vi "Loader.vi"(8 "error in (no error)":errorcluster, 10 "Path":path, 11 "Config_Read.lvclass":refnum<class "Config_Read_BML.lvclass">) -> (0 "error out":errorcluster, 1 "Pattern_Name":string, 2 "FRM_Data_Array":T1[](array[typedef]) {"Data" format="%x"; "Start_Addr" format="%x"}, 3 "Config_Read.lvclass out":refnum<class "Config_Read_BML.lvclass">)   [LabVIEW 2018, in "Config_Read_BML.lvclass"]
uses:
  Config_Read_BML.lvclass
  Frame_Data.ctl
  OperationMode.ctl
  BurstLength.ctl
  RW_Option.ctl
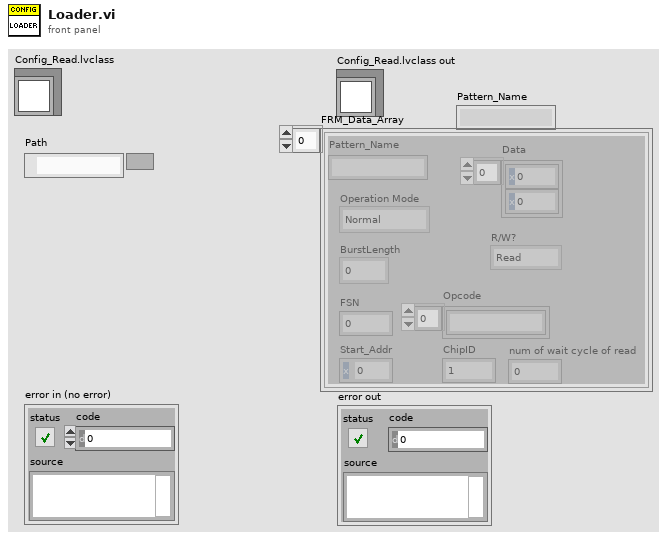
[diagram p1: front panel]
types:
  T1 = typedef "Config_Read_BML.lvclass/Frame_Data.ctl" = cluster{"Pattern_Name":string, "Operation Mode":T2, "BurstLength":T3, "FSN":u8, "Start_Addr":u16, "Data":u8[], "R/W?":T4, "Opcode":string[], "ChipID":u8, "num of wait cycle of read":i8}
  T2 = typedef "Config_Read_BML.lvclass/OperationMode.ctl" = enum8{"Normal", "ImmeEffect", "InitSlaveID", "LoadData"}
  T3 = typedef "Config_Read_BML.lvclass/BurstLength.ctl" = enum8{"0", "2", "3", "4", "5", "8", "16", "32"}
  T4 = typedef "Config_Read_BML.lvclass/RW_Option.ctl" = enum16{"Read", "Write", "R/W"}
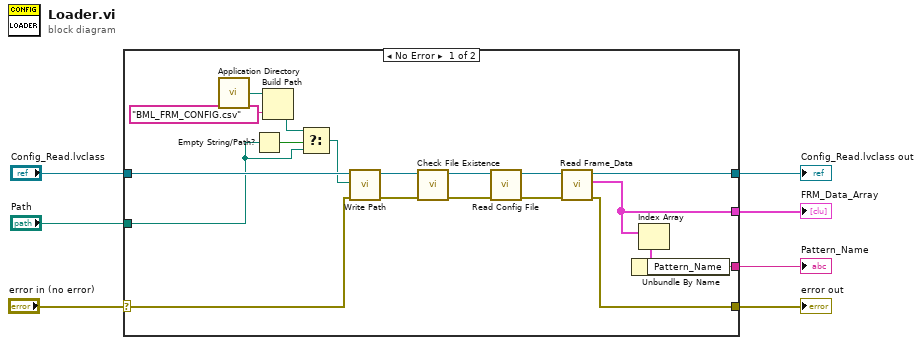
[diagram p0: block diagram]
diagram:
  n1 = case shown="No Error" "error in (no error)" {
    selector: "error in (no error)" -> [w15 w28]
    tunnel: "Config_Read.lvclass" -> [w26 w27]
    tunnel: "Path" -> [w24 _]
    tunnel: [w12 w27] -> w4
    tunnel: [w10 _] -> w2
    tunnel: [w11 w28] -> w3
    tunnel: [w8 _] -> w1
    frame No Error {
      n2 = call <vilib>:"Application Directory.vi"() -> ("Application Directory"=w22:path)
      n3 = Empty String/Path?(string/path=w24) -> (empty?=w25:bool)
      n4 = Build Path(base path=w22, name or relative path="BML_FRM_CONFIG.csv") -> (appended path=w20:path)
      n5 = Select(t=w20, s=w25, f=w24) -> (s? t:f=w23:path)
      n6 = call-dynamic "Write Path.vi"("error in (no error)"=w15, "Path"=w23, "Config_Read in"=w26) -> ("error out"=w18:errorcluster, "Config_Read out"=w19:refnum<class "Config_Read_BML.lvclass">)  [unwired: 7 in]
      n7 = call-dynamic "Check File Existence.vi"("error in (no error)"=w18, "Config_Read in"=w19) -> ("error out"=w16:errorcluster, "Config_Read out"=w17:refnum<class "Config_Read_BML.lvclass">)  [unwired: 8 in]
      n8 = call-dynamic "Read Config File.vi"("error in (no error)"=w16, "Config_Read in"=w17) -> ("error out"=w13:errorcluster, "Config_Read out"=w14:refnum<class "Config_Read_BML.lvclass">)  [unwired: 8 in]
      n9 = call-dynamic "Read Frame_Data.vi"("error in (no error)"=w13, "Config_Read in"=w14) -> ("error out"=w11:errorcluster, "FRM_Data_Array"=w10:T1[], "Config_Read out"=w12:refnum<class "Config_Read_BML.lvclass">)  [unwired: 7 in]
      n10 = Index Array(array=w10) -> (element=w9:T1)  [unwired: 1 in]
      n11 = Unbundle By Name(w9) -> ("Pattern_Name"=w8:string)
    }
    frame Error {
    }
  }
  "Config_Read.lvclass out" <- w4
  "error out" <- w3
  "FRM_Data_Array" <- w2
  "Pattern_Name" <- w1
